vi "Get Resource ID.vi"(11 "PWM in":refnum<class "PWM.lvclass">) -> (2 "Resource ID":string)   [LabVIEW 2020, in "CTI.lvlib" / "PWM.lvclass"]
uses:
  PWM.lvclass
  PWM.lvclass/PWM.ctl
  GPIO/GPIO.lvclass/GPIO.ctl
  GPIO/GPIO.lvclass
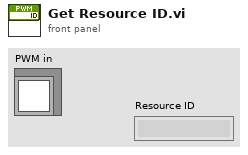
[diagram p1: front panel]
types:
  T1 = typedef "CTI.lvlib/GPIO Number.ctl" = i8
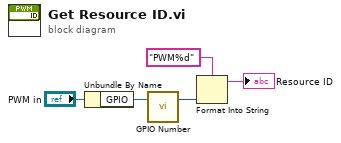
[diagram p0: block diagram]
diagram:
  n1 = Unbundle By Name("PWM in") -> ("GPIO"=w4:refnum<class "GPIO.lvclass">)
  n2 = call "GPIO Number.vi"("GPIO in"=w4) -> ("GPIO #"=w3:T1)  [unwired: 6 in]
  n3 = Format Into String(format string="PWM%d", w3) -> (resulting string=→"Resource ID":string)  [unwired: 2 in, 1 out]
